vi "Task05SubVI.vi"(11 "Array":bool[](array[boolean])) -> (3 "Numeric":u32)   [LabVIEW 2017]
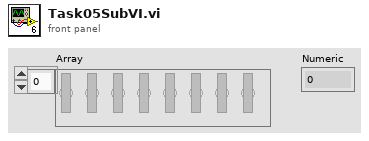
[diagram p1: front panel]
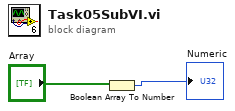
[diagram p0: block diagram]
diagram:
  n1 = Boolean Array To Number(Boolean array="Array") -> (number=→"Numeric":u32)
